vi "Output Rings.vi"() -> (1 "Text Ring":u16(ring)=2233 items=["Text Ring Value 1"=111, "Text Ring Value 2"=2233, "Text Ring Value 3"=4455, "Text Ring Value 4"=5566, "Text Ring Value 5"=7788], 2 "Menu Ring":i32(ring)=150 items=["Menu Item 1"=12, "Menu Item 2"=45, "Menu Item 3"=150, "Menu Item 4"=330, "Menu Item 5"=455], 3 "Enum":enum8{"AAA", "BBB", "CCCC", "DDDD", "EEEE"}(ring)=enum."CCCC")   [LabVIEW 2012]
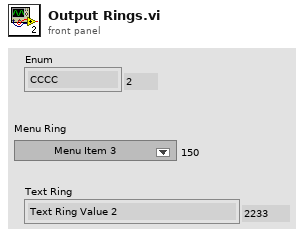
[diagram p1: front panel]
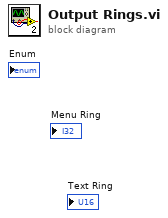
[diagram p0: block diagram]
diagram:
